vi "Constants.vi"() -> ()   [LabVIEW 2017, in "VeriStand Web Service Demo Shared.lvlib"]
doc: "Use this Global VI to access the GUIDs assigned to the page resources of the Custom Device."
uses:
  VeriStand Web Service Demo Shared.lvlib
panel:
  in  "Tab Control":enum32{"GUIDS", "Constants", "Properties"}(tab)
  in  "pg3":string="97a9f901-6a68-4174-8b54-51823094d7fd"
  in  "pg2":string="99731d0a-4c8d-4657-b35d-eee29e4cd168"
  in  "pg1":string="cda66537-2f45-42b8-9513-b9a32cfebcd0"
  in  "VeriStand Web Service Demo":string="ba752fcc-3ccd-45b5-9c7b-59b1f8d3942b"
  in  "Compiled.Settings":string="Compiled.Settings"
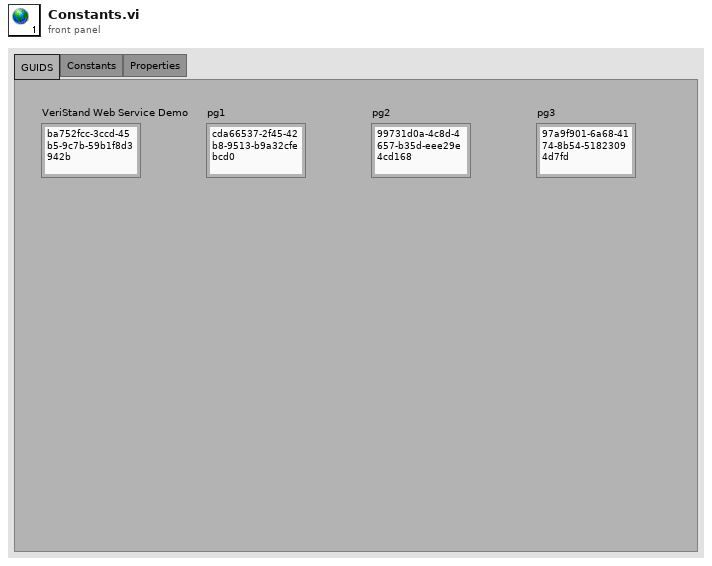
[diagram p1: front panel]
diagram:
